vi "Set and get merit factor array.vi"(7 "action":enum16{"set", "get", "initialise"}(ring)=enum."initialise", 8 "error in (no error)":errorcluster, 9 "array size":i32=5, 10 "merit factor":dbl, 11 "RSA in":refnum<class "RSA.lvclass">) -> (0 "error out":errorcluster, 1 "current merit factor":dbl, 2 "merit factor array":dbl[](array[numeric]), 3 "RSA out":refnum<class "RSA.lvclass">)   [LabVIEW 2012, in "RSA.lvclass"]
uses:
  RSA.lvclass
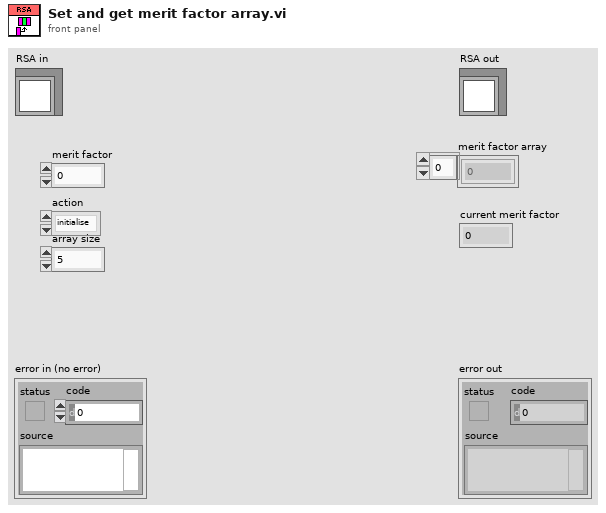
[diagram p1: front panel]
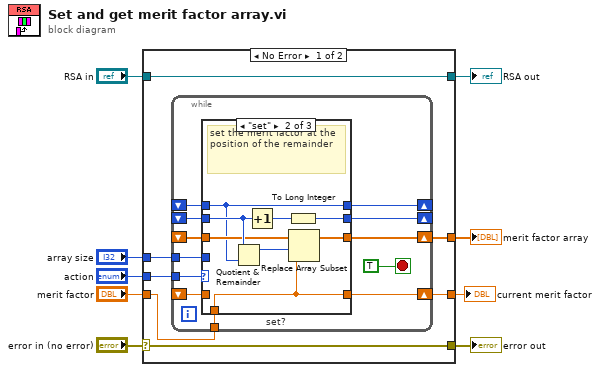
[diagram p0: block diagram]
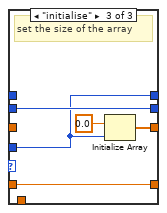
[diagram p3: hidden frame]
diagram:
  n1 = case shown="No Error" "error in (no error)" {
    selector: "error in (no error)" -> [w15 w47]
    tunnel: [w15 w47] -> w8
    tunnel: [w16 w46] -> w6
    tunnel: "RSA in" -> [w16 w46]
    tunnel: "merit factor" -> [w10 _]
    tunnel: "action" -> [w14 _]
    tunnel: [w13 _] -> w3
    tunnel: "array size" -> [w12 _]
    tunnel: [w11 _] -> w1
    frame No Error {
      n2 = while {
        shift-right: [w26] -> w13
        shift-left: _ -> [w23]
        shift-right: [w25] -> _
        shift-left: _ -> [w24]
        tunnel: w14 -> [w22]
        shift-right: [w20] -> _
        shift-left: _ -> [w21]
        tunnel: w12 -> [w19]
        shift-right: [w18] -> w11
        shift-left: _ -> [w27]
        tunnel: w10 -> [w17]
        stop <- TRUE stop-if-true
        n3 = case "set?" shown="\"set\"" w22 {
          tunnel: w27 -> [w29 _ w41]
          tunnel: [w31 w37 w42] -> w26
          tunnel: [w32 w35 w45] -> w25
          tunnel: w24 -> [w32 w40 w45]
          tunnel: w23 -> [w31 w38 _]
          tunnel: w21 -> [w30 w34 _]
          tunnel: [w30 w34 w43] -> w20
          tunnel: w19 -> [_ _ w43]
          tunnel: [w29 w33 w41] -> w18
          tunnel: w17 -> [_ w33 _]
          frame "get", Default {
            # "get the array"
          }
          frame "set" {
            # "set the merit factor at the position of the remainder"
            n4 = Quotient & Remainder(x=w40, y=w34) -> (x-y*floor(x/y)=w36:i32)  [unwired: 1 out]
            n5 = Increment(x=w40) -> (x+1=w39:i32)
            n6 = To Long Integer(number=w39) -> (32bit integer=w35:i32)
            n7 = Replace Array Subset(array=w38, new element=w33, index=w36) -> (w37:dbl[])
          }
          frame "initialise" {
            # "set the size of the array"
            n8 = Initialize Array(0.0 ("merit factor"), w43) -> (w42:dbl[])
          }
        }
      }
    }
    frame Error {
    }
  }
  "error out" <- w8
  "RSA out" <- w6
  "merit factor array" <- w3
  "current merit factor" <- w1
